vi "Stage 4.1 Adding Error Communication.vi"() -> ()   [LabVIEW 2020]
panel:
  out "Process Error":errorcluster
  out "error out":errorcluster
  out "error out Hardware":errorcluster
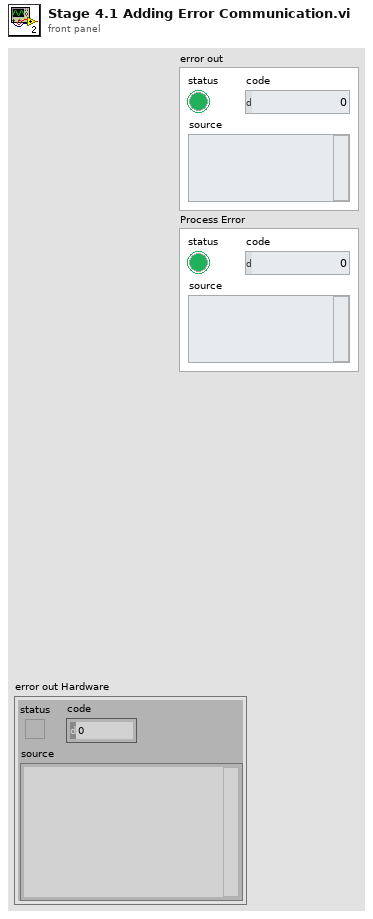
[diagram p1: front panel]
types:
  T1 = typedef "HRM-init_cluster.ctl" = cluster{"User events":T2}
  T2 = typedef "HRM-User_events.ctl" = cluster{"Signal to remove":refnum<user-event>, "Sample size":refnum<user-event>, "Filtered wf":refnum<user-event>, "Unfiltered wf":refnum<user-event>, "Raw wf":refnum<user-event>, "Pulse":refnum<user-event>, "stop":refnum<user-event>, "error msg":refnum<user-event>}
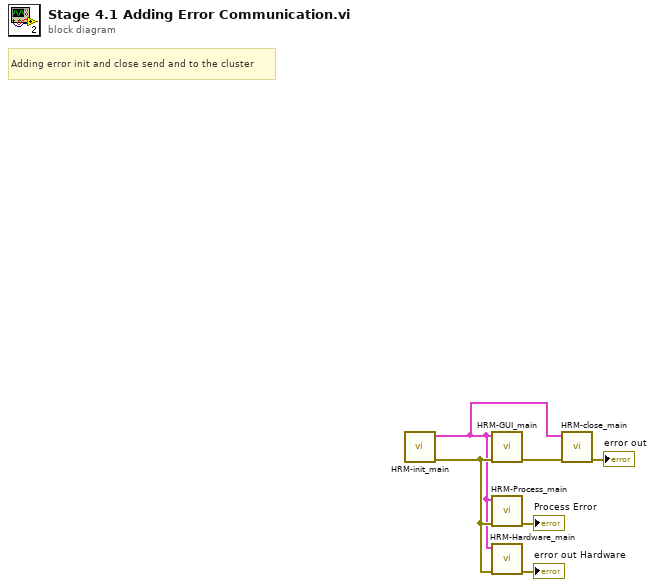
[diagram p0: block diagram]
diagram:
  # "Adding error init and close send and to the cluster"
  n1 = call "HRM-init_main.vi"() -> ("error out"=w3:errorcluster, "Init cluster"=w1:T1)  [unwired: 10 in]
  n2 = call "HRM-GUI_main.vi"("error in (no error)"=w3, "Init cluster"=w1) -> ("error out"=w2:errorcluster)  [unwired: 9 in]
  n3 = call "HRM-Process_main.vi"("error in (no error)"=w3, "Init cluster"=w1) -> ("error out"=→"Process Error":errorcluster)  [unwired: 9 in]
  n4 = call "HRM-Hardware_main.vi"("error in (no error)"=w3, "Init cluster"=w1) -> ("error out"=→"error out Hardware":errorcluster)  [unwired: 9 in]
  n5 = call "HRM-close_main.vi"("error in (no error)"=w2, "Init cluster"=w1) -> ("error out"=→"error out":errorcluster)  [unwired: 9 in]
